vi "Get State Value Index.vi"(8 "error in (no error)":errorcluster, 10 "State Value":dbl, 11 "Routing Channel Configuration":T1) -> (0 "error out":errorcluster, 3 "index":i32)   [LabVIEW 2020, in "Routing and Faulting Engine.lvlib"]
uses:
  Routing and Faulting Engine.lvlib
  Shared/Value-Connections Map.ctl
  Shared/Routing and Faulting Shared.lvlib
  Shared/Routing Channel Configuration.ctl
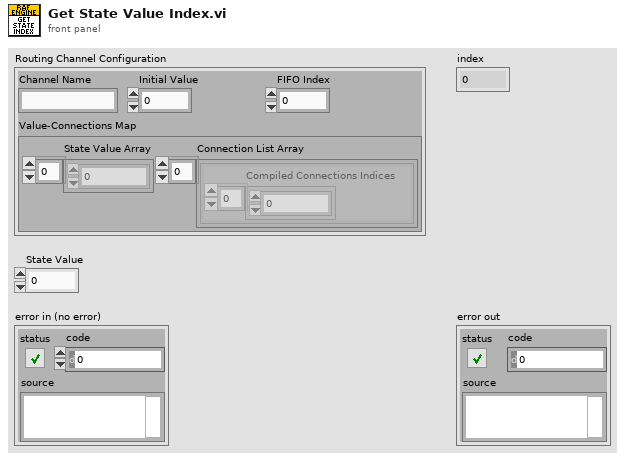
[diagram p1: front panel]
types:
  T1 = typedef "Routing and Faulting Shared.lvlib/Routing Channel Configuration.ctl" = cluster{"Channel Name":string, "Initial Value":dbl, "FIFO Index":i32, "Value-Connections Map":T2}
  T2 = typedef "Routing and Faulting Shared.lvlib/Value-Connections Map.ctl" = cluster{"State Value Array":i32[], "Connection List Array":cluster{"Compiled Connections Indices":i32[]}[]}
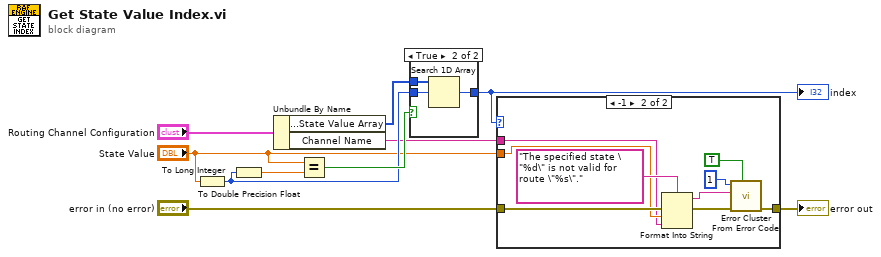
[diagram p0: block diagram]
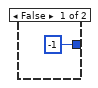
[diagram p3: hidden frame]
diagram:
  n1 = To Long Integer(number="State Value") -> (32bit integer=w7:i32)
  n2 = To Double Precision Float(number=w7) -> (double precision float=w6:dbl)
  n3 = Unbundle By Name("Routing Channel Configuration") -> ("Value-Connections Map.State Value Array"=w9:i32[], "Channel Name"=w1:string)
  n4 = Equal?(x="State Value", y=w6) -> (x = y?=w10:bool)
  n5 = case shown="True" w10 {
    tunnel: w7 -> [_ w14]
    tunnel: [-1 ("index of element") w12] -> w5
    tunnel: w9 -> [_ w13]
    frame False {
    }
    frame True {
      n6 = Search 1D Array(1D array=w13, element=w14) -> (index of element=w12:i32)  [unwired: 1 in]
    }
  }
  "index" <- w5
  n7 = case shown="-1" w5 {
    tunnel: "error in (no error)" -> [w15 w19]
    tunnel: [w15 w18] -> w3
    tunnel: "State Value" -> [_ w17]
    tunnel: w1 -> [_ w16]
    frame Default {
    }
    frame -1 {
      n8 = Format Into String(format string="The specified state \"%d\" is not valid for route \"%s\".", error in=w19, w17, w16) -> (resulting string=w23:string, error out=w22:errorcluster)  [unwired: 1 in]
      n9 = call <vilib>:"Error Cluster From Error Code.vi"("show call chain? (False)"=TRUE, "error in (no error)"=w22, "error message (\"\")"=w23, "error code (0)"=1) -> ("error out"=w18:errorcluster)  [unwired: 5 in]
    }
  }
  "error out" <- w3
